vi "Fast Channel Create FuncGlobal.vi"(0 "Parent Ref in":T1 format="%.0x", 1 "GUID (Default Channel)":string="03D3BB99-1485-13A6-561D1F898F032919", 2 "Action":enum16{"Open or Add", "Close Ref"}(ring), 3 "Highlight? (F)":bool, 5 "Channel Name":string, 7 "Channel":T2, 11 "error in (no error)":errorcluster, 12 "Property names":string[](array[string]), 13 "Property Values":variant[](array[variant])) -> (4 "Parent Ref out":T1 format="%.0x", 8 "Channel Ref":T1 format="%.0x", 15 "error out":errorcluster)   [LabVIEW 2011]
doc: "Creates an NI VeriStand Channel faster than the built in function does (when called in a loop). The built in function opens a reference and closes it within, causing it to be realllly slow in a loop. This functional global opens the reference on first call, but then saves it for later use.\n\nMake sure you close the refernce later."
uses:
  <vilib>/NI Veristand/Custom Device API/Custom Device Item Ref.ctl
  <vilib>/NI Veristand/Custom Device API/Custom Device Channel.ctl
  <vilib>/NI Veristand/Custom Device API/Custom Device Channel Type.ctl
  <vilib>/NI Veristand/Custom Device API/Custom Device API.lvlib
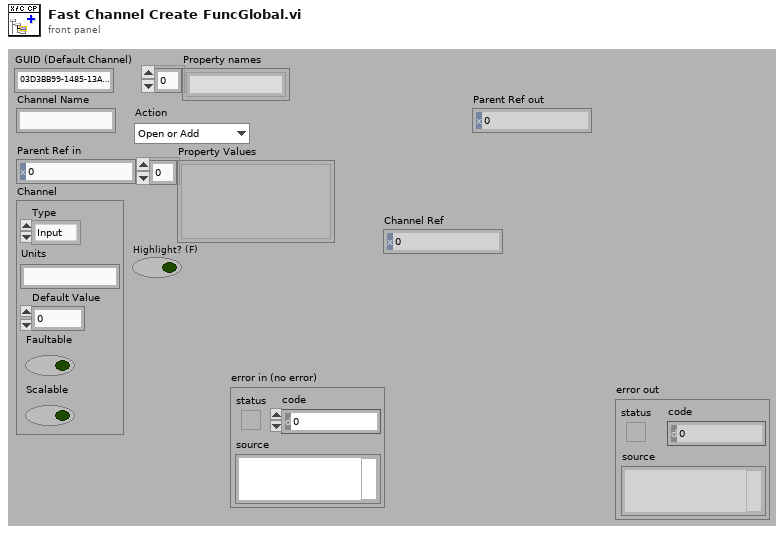
[diagram p1: front panel]
types:
  T1 = typedef "Custom Device API.lvlib/Custom Device Item Ref.ctl" = u64
  T2 = typedef "Custom Device API.lvlib/Custom Device Channel.ctl" = cluster{"Type":T3, "Units":string, "Default Value":dbl, "Faultable":bool, "Scalable":bool}
  T3 = typedef "Custom Device API.lvlib/Custom Device Channel Type.ctl" = enum16{"Input", "Output"}
  T4 = typedef "Custom Devices Storage.lvlib/Custom Device Item Ref.ctl" = u64
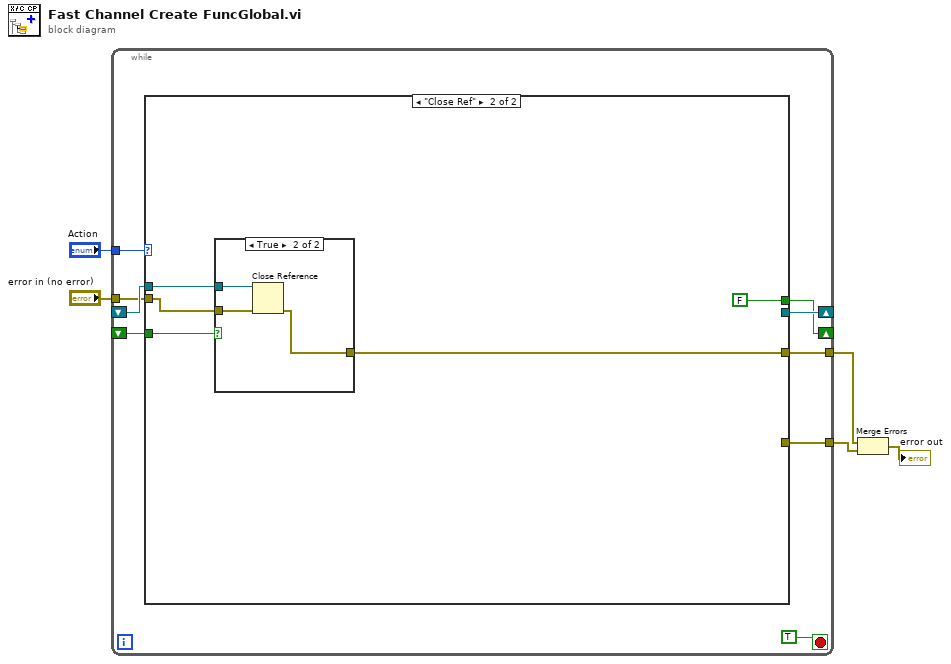
[diagram p0: block diagram]
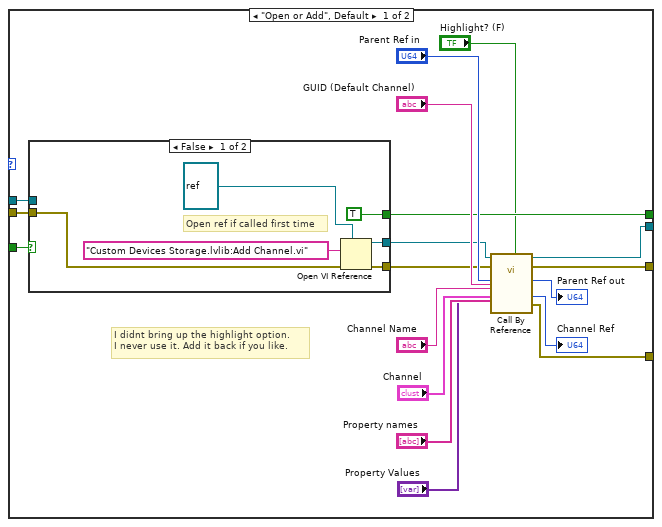
[diagram p2: hidden frame]
diagram:
  n1 = while {
    tunnel: "Action" -> [w14]
    shift-right: [w13] -> _
    shift-left: _ -> [w12]
    tunnel: "error in (no error)" -> [w11]
    tunnel: [w10] -> w2
    tunnel: [w9] -> w1
    shift-right: [w8] -> _
    shift-left: _ -> [w7]
    stop <- TRUE stop-if-true
    n2 = case shown="\"Close Ref\"" w14 {
      tunnel: w12 -> [w16 w46]
      tunnel: [w24 _] -> w13
      tunnel: w11 -> [w21 w45]
      tunnel: [w23 _] -> w10
      tunnel: [w22 w42] -> w9
      tunnel: [w19 FALSE] -> w8
      tunnel: w7 -> [w18 w43]
      frame "Open or Add", Default {
        # "I didnt bring up the highlight option.\nI never use it. Add it back if you like."
        n3 = case shown="False" w18 {
          selector: w18 -> [_ w39]
          tunnel: w21 -> [w36 w40]
          tunnel: [w35 w40] -> w20
          tunnel: [TRUE w39] -> w19
          tunnel: [w33 w41] -> w17
          tunnel: w16 -> [_ w41]
          frame False {
            # "Open ref if called first time"
            n4 = Open VI Reference(type specifier VI Refnum (for type only)=refnum<vi> refnum, vi path="Custom Devices Storage.lvlib:Add Channel.vi", error in (no error)=w36) -> (vi reference=w33:refnum<vi>, error out=w35:errorcluster)  [unwired: 1 in, 2 out]
          }
          frame True {
            # "Don't open the ref if already open"
          }
        }
        n5 = call-by-ref "?"(reference=w17, error in=w20, "Property Values"="Property Values", "Highlight? (F)"="Highlight? (F)", "Property names"="Property names", "GUID (Default Channel)"="GUID (Default Channel)", "Channel"="Channel", "Channel Name"="Channel Name", "Parent Ref in"="Parent Ref in") -> (reference out=w24:refnum<vi>, error out=w22:errorcluster, 0:"error out"=w23:errorcluster, "Channel Ref"=→"Channel Ref":T4, "Parent Ref out"=→"Parent Ref out":T1)  [unwired: 2 in]
      }
      frame "Close Ref" {
        n6 = case shown="True" w43 {
          tunnel: w46 -> [_ w50]
          tunnel: w45 -> [w47 w49]
          tunnel: [w47 w48] -> w42
          frame False {
          }
          frame True {
            n7 = Close Reference(reference=w50, error in (no error)=w49) -> (error out=w48:errorcluster)
          }
        }
      }
    }
  }
  n8 = Merge Errors(w1, w2) -> (→"error out":errorcluster)
